vi "ReadRecords.vi"(8 "error in (no error)":errorcluster, 10 "Num records to read":i32, 11 "FpgaRef5782 in":refnum<class "FpgaRef5782.lvclass">) -> (0 "error out":errorcluster, 2 "Data":dbl[][](array[numeric]), 3 "FpgaRef5782 out":refnum<class "FpgaRef5782.lvclass">)   [LabVIEW 2018, in "FpgaRef5782.lvclass"]
uses:
  FpgaRef5782.lvclass
  FpgaRef5782.lvclass/FpgaRef5782.ctl
  <vilib>/Utility/error.llb/Error Cluster From Error Code.vi
  <vilib>/rvi/errors/niLvFpgaAdjustHostInterfaceError.vi
  <vilib>/rvi/interface/nirviMethod/nirviMethod.xnode
  5782 FPGA ref.ctl
  <vilib>/FPGAPlugInAG/Dynamic/niLvFpga_ReadFifo_Dynamic.vi
  <vilib>/rvi/errors/niLvFpgaMergeErrorWithErrorCode.vi
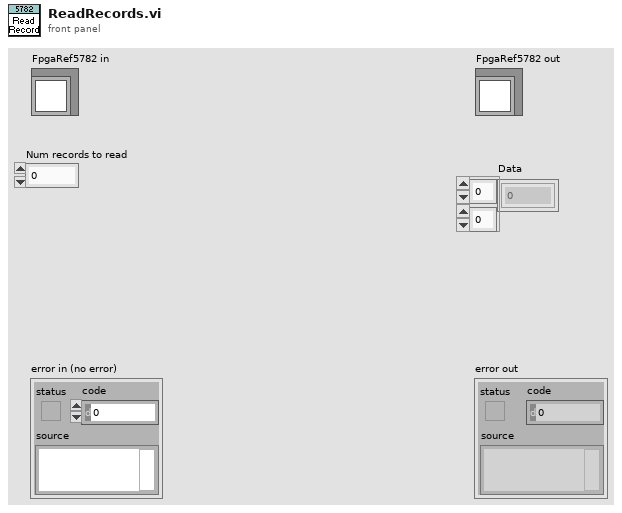
[diagram p1: front panel]
types:
  T1 = typedef "5782 FPGA ref.ctl" = refnum<k20>
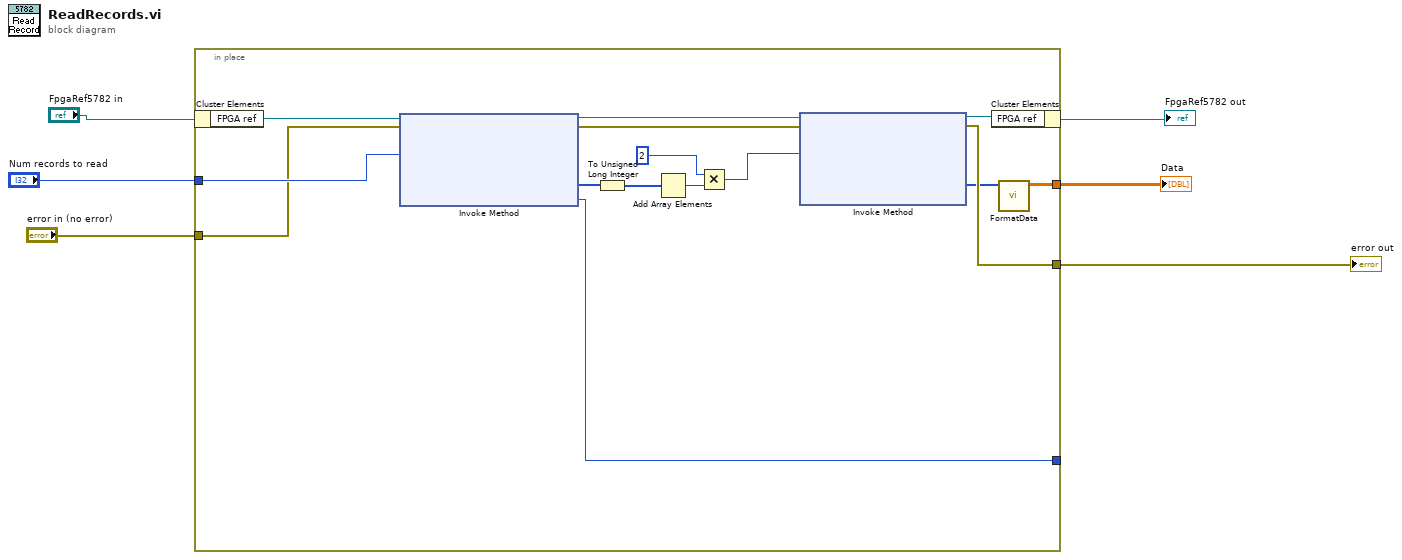
[diagram p0: block diagram]
diagram:
  n1 = in-place {
    in-place-border: "Num records to read" -> [w20]
    in-place-border: "error in (no error)" -> [w19]
    in-place-border: [w11] -> w2
    in-place-border: [w9] -> w1
    in-place-border: [w8] -> _
    n2 = in-place-cluster #1("FpgaRef5782 in") -> ("FPGA ref"=w21:T1)
    n3 = xnode "Invoke Method"("FPGA VI Reference In"=w21, "error in"=w19, "Number of Elements"=w20) -> ("FPGA VI Reference Out"=w14:T1, "error out"=w10:errorcluster, "Data"=w18:u16[], "Elements Remaining"=w8:u32)  [unwired: 1 in]
    n4 = To Unsigned Long Integer(number=w18) -> (unsigned 32bit integer=w17:u32[])
    n5 = Add Array Elements(numeric array=w17) -> (sum=w16:u32)
    n6 = Multiply(x=u32 2, y=w16) -> (x*y=w13:u32)
    n7 = xnode "Invoke Method"("FPGA VI Reference In"=w14, "error in"=w10, "Number of Elements"=w13) -> ("FPGA VI Reference Out"=w12:T1, "error out"=w9:errorcluster, "Data"=w7:u64[])  [unwired: 1 in, 1 out]
    n8 = in-place-cluster #1("FPGA ref"=w12) -> (→"FpgaRef5782 out":refnum<class "FpgaRef5782.lvclass">)
    n9 = call "FormatData.vi"("Raw data"=w7) -> ("Scaled"=w11:dbl[][])  [unwired: 10 in]
  }
  "error out" <- w1
  "Data" <- w2
